vi "UpdateValueConfig.vi"(8 "error in (no error)":errorcluster, 10 "McodeConfigNumber":dbl, 11 "XuLyStringUART in":refnum<class "XuLyStringUART.lvclass">) -> (0 "error out":errorcluster, 3 "XuLyStringUART out":refnum<class "XuLyStringUART.lvclass">)   [LabVIEW 2014, in "LibraryGcode.lvlib" / "XuLyStringUART.lvclass"]
uses:
  XuLyStringUART.lvclass
  ListMcodeConfig.ctl
  XuLyStringUART.lvclass/XuLyStringUART.ctl
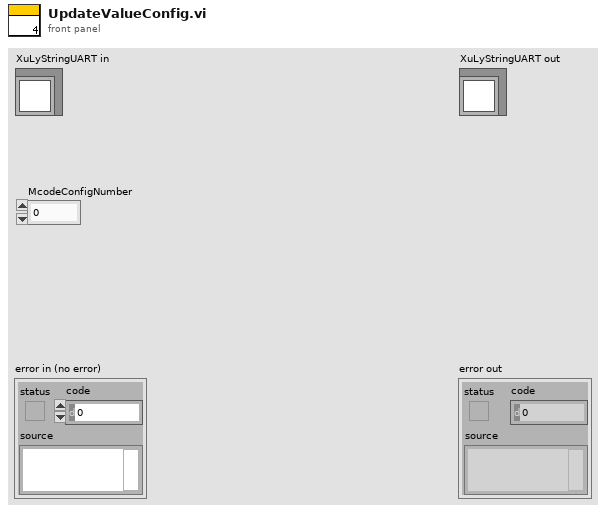
[diagram p1: front panel]
types:
  T1 = typedef "LibraryGcode.lvlib/XuLyStringUART.lvclass/ListMcodeConfig.ctl" = enum16{"M203", "M201", "M92", "M3001", "M204"}
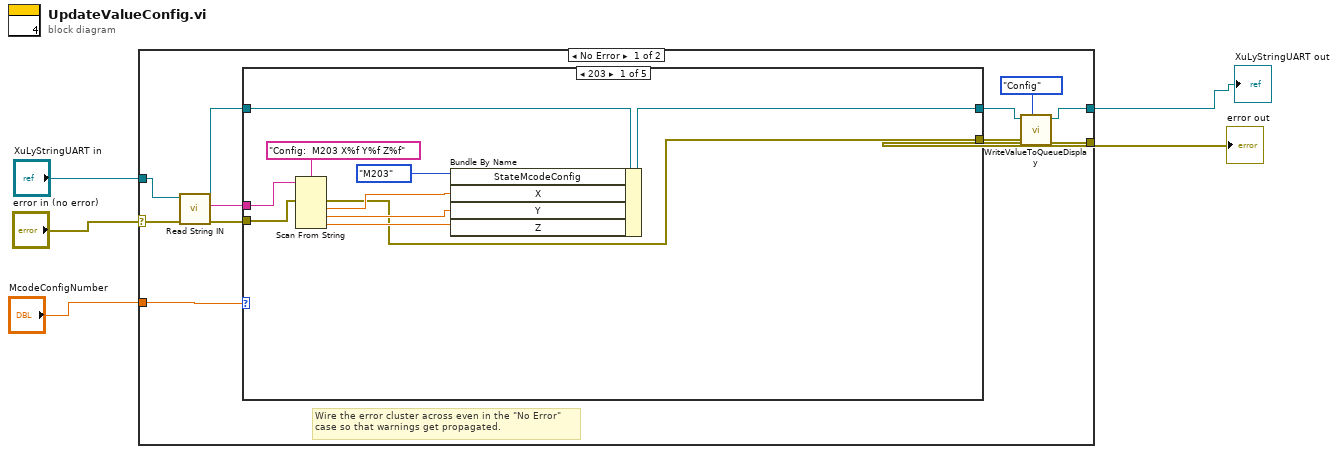
[diagram p0: block diagram]
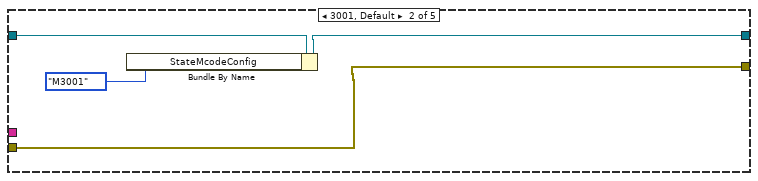
[diagram p2: hidden frame]
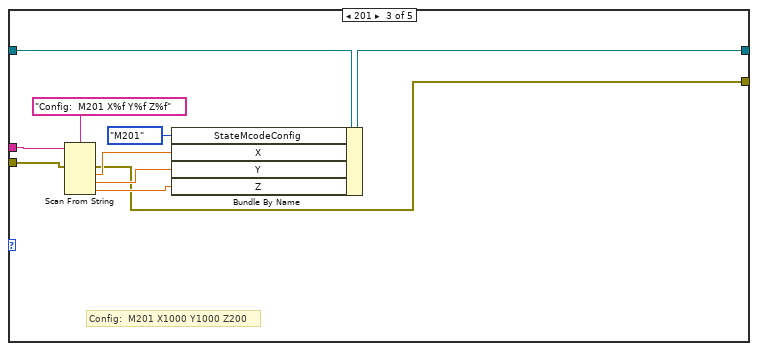
[diagram p3: hidden frame]
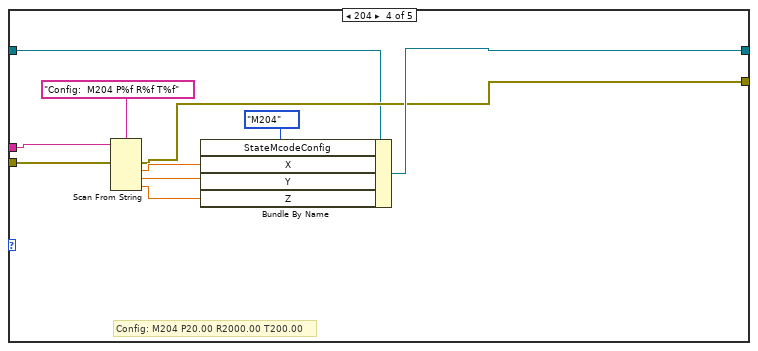
[diagram p4: hidden frame]
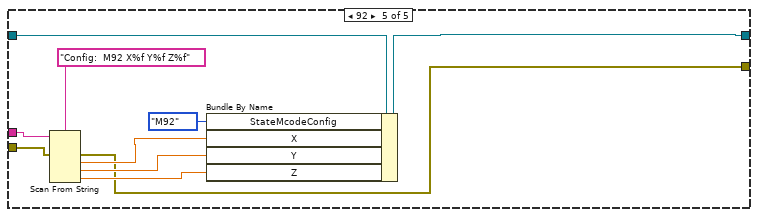
[diagram p5: hidden frame]
diagram:
  n1 = case shown="No Error" "error in (no error)" {
    selector: "error in (no error)" -> [w11 w62]
    tunnel: [w8 w62] -> w4
    tunnel: [w7 w61] -> w1
    tunnel: "XuLyStringUART in" -> [w15 w61]
    tunnel: "McodeConfigNumber" -> [w16 _]
    frame No Error {
      # "Wire the error cluster across even in the \"No Error\"\ncase so that warnings get propagated."
      n2 = call-dynamic "Read String IN.vi"("error in (no error)"=w11, "XuLyStringUART in"=w15) -> ("error out"=w12:errorcluster, "String IN"=w13:string, "XuLyStringUART out"=w14:refnum<class "XuLyStringUART.lvclass">)  [unwired: 7 in]
      n3 = case shown="203" w16 {
        tunnel: w14 -> [w24 w30 w37 w41 w58]
        tunnel: [w23 w28 w36 w49 w51] -> w10
        tunnel: w12 -> [w25 w27 w39 w44 w59]
        tunnel: [w18 w27 w31 w43 w53] -> w9
        tunnel: w13 -> [w17 _ w38 w42 w52]
        frame 203 {
          n4 = Scan From String(format string="Config:  M203 X%f Y%f Z%f", input string=w17, error in=w25) -> (error out=w18:errorcluster, output 1=w21:dbl, output 2=w20:dbl, output 3=w19:dbl)  [unwired: 4 in, 2 out]
          n5 = Bundle By Name(cluster=w24, "StateMcodeConfig"=ListMcodeConfig."M203" ("OUTCONFIG.StateMcodeConfig"), "X"=w21, "Y"=w20, "Z"=w19) -> (w23:refnum<class "XuLyStringUART.lvclass">)
        }
        frame 3001, Default {
          n6 = Bundle By Name(cluster=w30, "StateMcodeConfig"=ListMcodeConfig."M3001" ("OUTCONFIG.StateMcodeConfig")) -> (w28:refnum<class "XuLyStringUART.lvclass">)
        }
        frame 201 {
          # "Config:  M201 X1000 Y1000 Z200"
          n7 = Scan From String(format string="Config:  M201 X%f Y%f Z%f", input string=w38, error in=w39) -> (error out=w31:errorcluster, output 1=w35:dbl, output 2=w34:dbl, output 3=w33:dbl)  [unwired: 4 in, 2 out]
          n8 = Bundle By Name(cluster=w37, "StateMcodeConfig"=ListMcodeConfig."M201" ("OUTCONFIG.StateMcodeConfig"), "X"=w35, "Y"=w34, "Z"=w33) -> (w36:refnum<class "XuLyStringUART.lvclass">)
        }
        frame 204 {
          # "Config: M204 P20.00 R2000.00 T200.00"
          n9 = Scan From String(format string="Config:  M204 P%f R%f T%f", input string=w42, error in=w44) -> (error out=w43:errorcluster, output 1=w47:dbl, output 2=w45:dbl, output 3=w46:dbl)  [unwired: 4 in, 2 out]
          n10 = Bundle By Name(cluster=w41, "StateMcodeConfig"=ListMcodeConfig."M204" ("OUTCONFIG.StateMcodeConfig"), "X"=w47, "Y"=w45, "Z"=w46) -> (w49:refnum<class "XuLyStringUART.lvclass">)
        }
        frame 92 {
          n11 = Scan From String(format string="Config:  M92 X%f Y%f Z%f", input string=w52, error in=w59) -> (error out=w53:errorcluster, output 1=w56:dbl, output 2=w55:dbl, output 3=w54:dbl)  [unwired: 4 in, 2 out]
          n12 = Bundle By Name(cluster=w58, "StateMcodeConfig"=ListMcodeConfig."M92" ("OUTCONFIG.StateMcodeConfig"), "X"=w56, "Y"=w55, "Z"=w54) -> (w51:refnum<class "XuLyStringUART.lvclass">)
        }
      }
      n13 = call-dynamic "WriteValueToQueueDisplay.vi"("XuLyStringUART in"=w10, "error in (no error)"=w9, "Writepara"=enum16{"Config", "Pos"}."Config") -> ("XuLyStringUART out"=w7:refnum<class "XuLyStringUART.lvclass">, "error out"=w8:errorcluster)  [unwired: 6 in]
    }
    frame Error {
    }
  }
  "error out" <- w4
  "XuLyStringUART out" <- w1
